vi "New Read.vi"(0 "Process_REF":string="Temperature", 1 "physical channels":tag) -> ()   [LabVIEW 2018]
uses:
  <vilib>/DAQmx/read.llb/DAQmx Read (Analog 1D DBL NChan 1Samp).vi
  <vilib>/DAQmx/create/channels.llb/DAQmx Create Channel (AI-Temperature-Thermocouple).vi
  <vilib>/DAQmx/miscellaneous.llb/DAQmx Fill In Error Info.vi
panel:
  in  "Abort":bool
  out "error out":errorcluster
  in  "error in (no error)":errorcluster
  out "Thermocouple 5":dbl
  out "Thermocouple 3":dbl
  out "Thermocouple 4":dbl
  out "Thermocouple 2":dbl
  out "Thermocouple 1":dbl
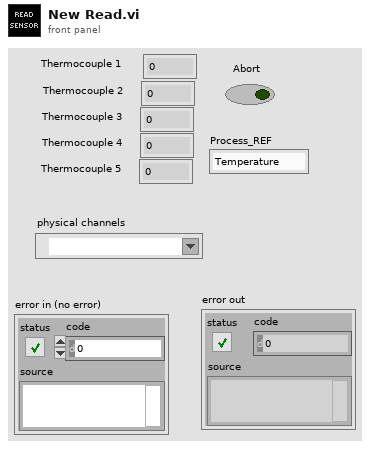
[diagram p1: front panel]
types:
  T1 = cluster{"data[0]":dbl, "data[1]":dbl, "data[2]":dbl, "data[3]":dbl, "data[4]":dbl}
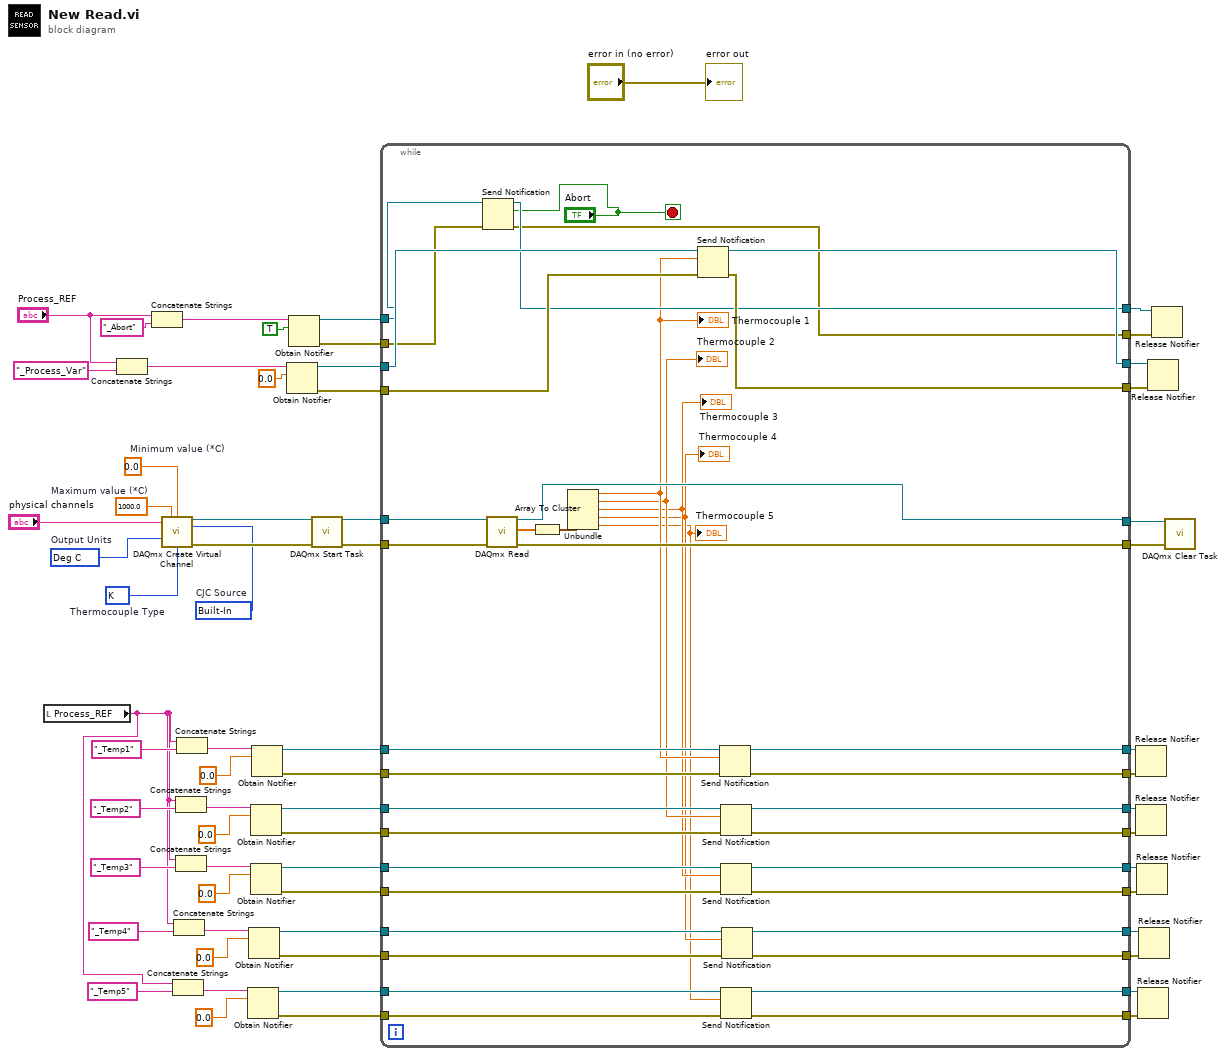
[diagram p0: block diagram]
diagram:
  w59 = 10143 items=["Deg C"=10143, "Deg F"=10144, "Kelvins"=10325, "Deg R"=10145, "From Custom Scale"=10065]  # Output Units
  w62 = 10073 items=["J"=10072, "K"=10073, "N"=10077, "R"=10082, "S"=10085, "T"=10086, "B"=10047, "E"=10055]  # Thermocouple Type
  w60 = 1000.0  # Maximum value (*C)
  w61 = 0.0  # Minimum value (*C)
  w58 = 10200 items=["Built-In"=10200, "Constant Value"=10116, "Channel"=10113]  # CJC Source
  n1 = local read "Process_REF"() -> (w2:string)
  n2 = Concatenate Strings("Process_REF", "_Process_Var" ("name (unnamed)")) -> (w40:string)
  n3 = Concatenate Strings("Process_REF", "_Abort") -> (w39:string)
  n4 = call-poly <vilib>:"DAQmx Create Virtual Channel.vi"("maximum value"=w60, "minimum value"=w61, "physical channels"="physical channels", "cjc source"=w58, "units"=w59, "thermocouple type"=w62) -> ("task out"=w64:refnum<k21>, "error out"=w63:errorcluster)  [unwired: 8 in]
  n5 = Concatenate Strings(w2, "_Temp5") -> (w20:string)
  n6 = Concatenate Strings(w2, "_Temp4") -> (w23:string)
  n7 = Concatenate Strings(w2, "_Temp2") -> (w29:string)
  n8 = Concatenate Strings(w2, "_Temp3") -> (w26:string)
  n9 = Concatenate Strings(w2, "_Temp1") -> (w36:string)
  n10 = Obtain Notifier(name (unnamed)=w20, notification data type=0.0) -> (notifier out=w15:refnum<notifier>, error out=w12:errorcluster)  [unwired: 2 in, 1 out]
  n11 = Obtain Notifier(name (unnamed)=w23, notification data type=0.0) -> (notifier out=w16:refnum<notifier>, error out=w11:errorcluster)  [unwired: 2 in, 1 out]
  n12 = Obtain Notifier(name (unnamed)=w29, notification data type=0.0) -> (notifier out=w18:refnum<notifier>, error out=w14:errorcluster)  [unwired: 2 in, 1 out]
  n13 = Obtain Notifier(name (unnamed)=w26, notification data type=0.0) -> (notifier out=w17:refnum<notifier>, error out=w13:errorcluster)  [unwired: 2 in, 1 out]
  n14 = Obtain Notifier(name (unnamed)=w36, notification data type=0.0) -> (notifier out=w34:refnum<notifier>, error out=w32:errorcluster)  [unwired: 2 in, 1 out]
  n15 = Obtain Notifier(name (unnamed)=w40, notification data type=0.0) -> (notifier out=w52:refnum<notifier>, error out=w51:errorcluster)  [unwired: 2 in, 1 out]
  n16 = Obtain Notifier(name (unnamed)=w39, notification data type=TRUE) -> (notifier out=w48:refnum<notifier>, error out=w47:errorcluster)  [unwired: 2 in, 1 out]
  n17 = call <vilib>:"DAQmx Start Task.vi"("task/channels in"=w64, "error in"=w63) -> ("task out"=w56:refnum<k21>, "error out"=w55:errorcluster)  [unwired: 12 in]
  n18 = while {
    tunnel: w56 -> [w104]
    tunnel: w55 -> [w103]
    tunnel: [w102] -> w54
    tunnel: [w101] -> w53
    tunnel: w52 -> [w100]
    tunnel: w51 -> [w99]
    tunnel: [w98] -> w50
    tunnel: [w97] -> w49
    tunnel: w48 -> [w96]
    tunnel: w47 -> [w93]
    tunnel: [w95] -> w46
    tunnel: [w94] -> w45
    tunnel: [w88] -> w33
    tunnel: w34 -> [w89]
    tunnel: w32 -> [w87]
    tunnel: [w86] -> w31
    tunnel: w18 -> [w83]
    tunnel: w17 -> [w84]
    tunnel: w16 -> [w82]
    tunnel: w15 -> [w85]
    tunnel: [w81] -> w4
    tunnel: w14 -> [w80]
    tunnel: w13 -> [w79]
    tunnel: w12 -> [w78]
    tunnel: w11 -> [w77]
    tunnel: [w76] -> w3
    tunnel: [w75] -> w5
    tunnel: [w74] -> w6
    tunnel: [w73] -> w8
    tunnel: [w72] -> w7
    tunnel: [w71] -> w10
    tunnel: [w70] -> w9
    stop <- "Abort" stop-if-true
    n19 = Send Notification(notification="Abort", notifier=w96, error in (no error)=w93) -> (notifier out=w95:refnum<notifier>, error out=w94:errorcluster)
    n20 = call-poly <vilib>:"DAQmx Read.vi"("task/channels in"=w104, "error in"=w103) -> ("task out"=w102:refnum<k21>, "data"=w91:dbl[], "error out"=w101:errorcluster)  [unwired: 11 in]
    n21 = Array To Cluster(array=w91) -> (cluster=w90:T1)
    n22 = Unbundle(w90) -> ("data[0]"=w69:dbl, "data[1]"=w68:dbl, "data[2]"=w67:dbl, "data[3]"=w66:dbl, "data[4]"=w65:dbl)
    "Thermocouple 1" <- w69
    "Thermocouple 2" <- w68
    "Thermocouple 3" <- w67
    "Thermocouple 4" <- w66
    "Thermocouple 5" <- w65
    n23 = Send Notification(notification=w69, notifier=w100, error in (no error)=w99) -> (notifier out=w98:refnum<notifier>, error out=w97:errorcluster)
    n24 = Send Notification(notification=w69, notifier=w89, error in (no error)=w87) -> (notifier out=w88:refnum<notifier>, error out=w86:errorcluster)
    n25 = Send Notification(notification=w68, notifier=w83, error in (no error)=w80) -> (notifier out=w81:refnum<notifier>, error out=w76:errorcluster)
    n26 = Send Notification(notification=w67, notifier=w84, error in (no error)=w79) -> (notifier out=w74:refnum<notifier>, error out=w75:errorcluster)
    n27 = Send Notification(notification=w65, notifier=w85, error in (no error)=w78) -> (notifier out=w71:refnum<notifier>, error out=w70:errorcluster)
    n28 = Send Notification(notification=w66, notifier=w82, error in (no error)=w77) -> (notifier out=w73:refnum<notifier>, error out=w72:errorcluster)
  }
  n29 = Release Notifier(notifier=w33, error in (no error)=w31) -> ()  [unwired: 1 in, 3 out]
  n30 = Release Notifier(notifier=w4, error in (no error)=w3) -> ()  [unwired: 1 in, 3 out]
  n31 = Release Notifier(notifier=w6, error in (no error)=w5) -> ()  [unwired: 1 in, 3 out]
  n32 = Release Notifier(notifier=w10, error in (no error)=w9) -> ()  [unwired: 1 in, 3 out]
  n33 = Release Notifier(notifier=w8, error in (no error)=w7) -> ()  [unwired: 1 in, 3 out]
  n34 = Release Notifier(notifier=w50, error in (no error)=w49) -> ()  [unwired: 1 in, 3 out]
  n35 = Release Notifier(notifier=w46, error in (no error)=w45) -> ()  [unwired: 1 in, 3 out]
  n36 = call <vilib>:"DAQmx Clear Task.vi"("task in"=w54, "error in"=w53) -> ()  [unwired: 13 in, 1 out]
  "error out" <- "error in (no error)"
